vi "Delete_with_Check.vi"(1 "FilePath":path) -> (0 "Deleted Filepath":path)   [LabVIEW 2010]
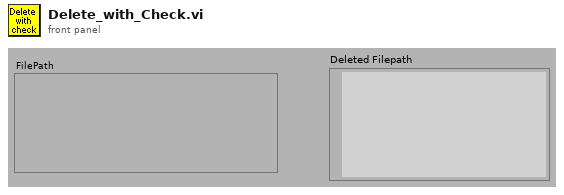
[diagram p1: front panel]
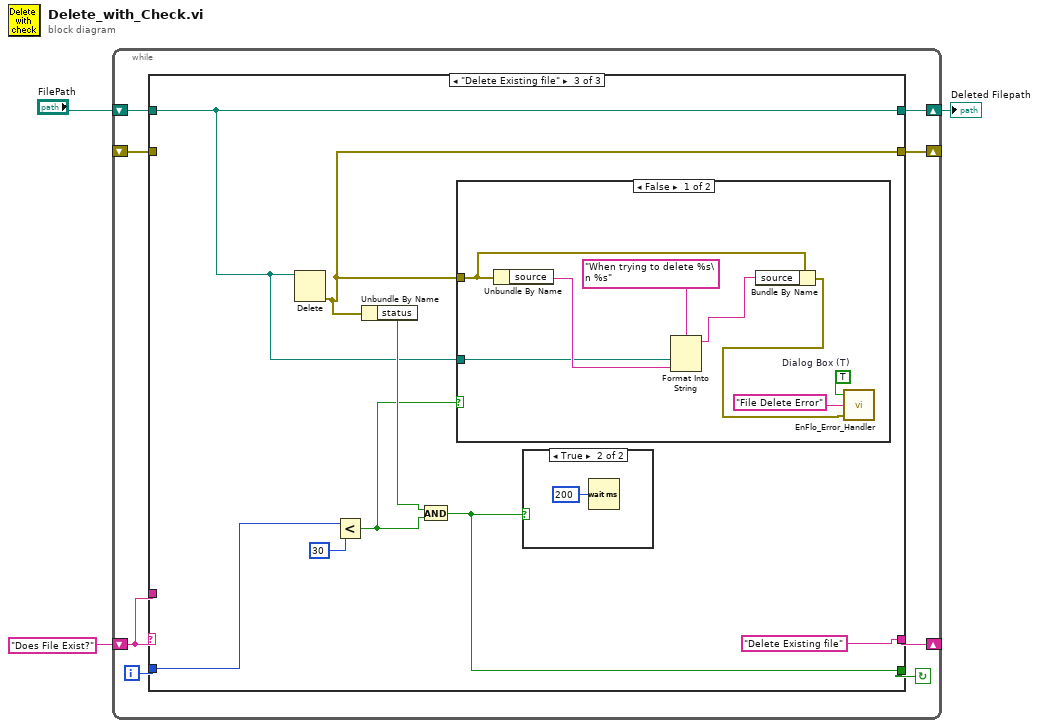
[diagram p0: block diagram]
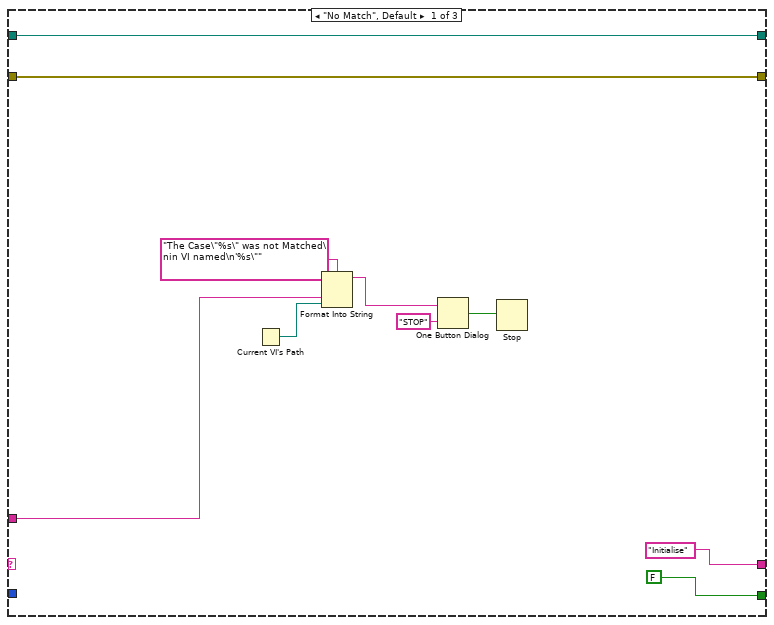
[diagram p2: hidden frame]
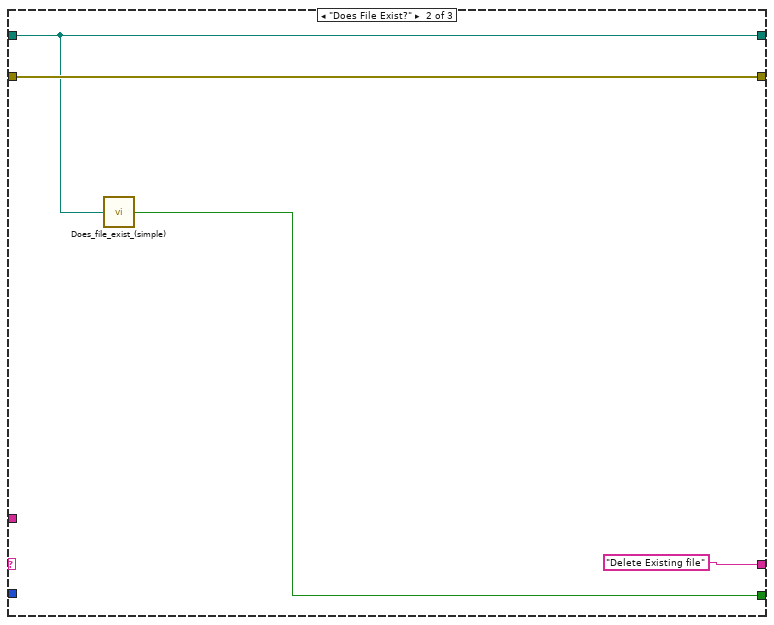
[diagram p3: hidden frame]
diagram:
  n1 = while {
    shift-left: "Does File Exist?" -> [w9]
    shift-right: [w10] -> _
    shift-right: [w7] -> w1
    shift-left: "FilePath" -> [w8]
    shift-right: [w6] -> _
    shift-left: _ -> [w5]
    i -> [w4]
    stop <- w11 continue-if-true
    n2 = case shown="\"Delete Existing file\"" w9 {
      tunnel: [FALSE w22 w26] -> w11
      tunnel: ["Initialise" "Delete Existing file" ("t") "Delete Existing file" ("t")] -> w10
      tunnel: w9 -> [w16 _ _]
      tunnel: w8 -> [w13 w24 w28]
      tunnel: [w13 w24 w28] -> w7
      tunnel: [w12 w25 w29] -> w6
      tunnel: w5 -> [w12 w25 _]
      tunnel: w4 -> [_ _ w32]
      frame "No Match", Default {
        n3 = Current VI's Path() -> (path=w15:path)
        n4 = Format Into String(format string="The Case\"%s\" was not Matched\nin VI named\n'%s\"" ("Format String"), w16, w15) -> (resulting string=w19:string)  [unwired: 2 in, 1 out]
        n5 = One Button Dialog(message=w19, button name ("OK")="STOP") -> (true=w17:bool)
        n6 = Stop(stop? (T)=w17) -> ()
      }
      frame "Does File Exist?" {
        n7 = call "Does_file_exist_(simple).vi"("Pathname"=w24) -> ("exists?"=w22:bool)
      }
      frame "Delete Existing file" {
        n8 = Delete(path (use dialog)=w28) -> (error out=w29:errorcluster)  [unwired: 1 in, 5 out]
        n9 = Less?(x=w32, y=30) -> (x < y?=w30:bool)
        n10 = Unbundle By Name(w29) -> ("status"=w31:bool)
        n11 = And(x=w31, y=w30) -> (x .and. y?=w26:bool)
        n12 = case shown="False" w30 {
          tunnel: w29 -> [w37 _]
          tunnel: w28 -> [w38 _]
          frame False {
            w36 = TRUE  # Dialog Box (T)
            n13 = Unbundle By Name(w37) -> ("source"=w41:string)
            n14 = Format Into String(format string="When trying to delete %s\n %s", w38, w41) -> (resulting string=w39:string)  [unwired: 2 in, 1 out]
            n15 = Bundle By Name(cluster=w37, "source"=w39) -> (w34:errorcluster)
            n16 = call "EnFlo_Error_Handler.vi"("error in (no error)"=w34, "Error Type"="File Delete Error", "Dialog Box (T)"=w36) -> ()  [unwired: 3 out]
          }
          frame True {
          }
        }
        n17 = case shown="True" w26 {
          frame False {
          }
          frame True {
            n18 = Wait (ms)(milliseconds to wait=u32 200) -> ()  [unwired: 1 out]
          }
        }
      }
    }
  }
  "Deleted Filepath" <- w1
